vi "Initialiser caméra_CP.vi"(8 "entrée d'erreur (pas d'erreur)":errorcluster) -> (0 "sortie d'erreur":errorcluster, 2 "Camera":refnum<class "Camera.lvclass">, 3 "Buffer en sortie":refnum<class "Buffer.lvclass">, 4 "Devices":T1[](array[typedef]), 5 "Pixel Formats":string[](array[string]), 7 "Pixel Format":string)   [LabVIEW 2026]
uses:
  <vilib>/Serenial/G Industrial Camera/g_industrial_cam/Device Enumeration.ctl
  <vilib>/Serenial/G Industrial Camera/g_industrial_cam/Camera/Camera.lvclass
  <vilib>/Serenial/G Industrial Camera/g_industrial_cam/Buffer/Buffer.lvclass
  <vilib>/Serenial/G Industrial Camera/g_industrial_cam/Camera/Camera.lvclass/Camera.ctl
  <vilib>/Serenial/G Industrial Camera/g_industrial_cam/Buffer/Buffer.lvclass/Buffer.ctl
  <vilib>/Serenial/G Industrial Camera/g_industrial_cam/Camera/GetSetPixelFormat.vi
  <vilib>/Serenial/G Industrial Camera/g_industrial_cam/Camera/Check Not Disconnected.vi
  <vilib>/Utility/error.llb/Error Cluster From Error Code.vi
  <vilib>/Serenial/G Industrial Camera/g_industrial_cam/Camera/Destroy Stream Events.vi
  <vilib>/Serenial/G Industrial Camera/g_industrial_cam/g_industrial_cam.lvlib
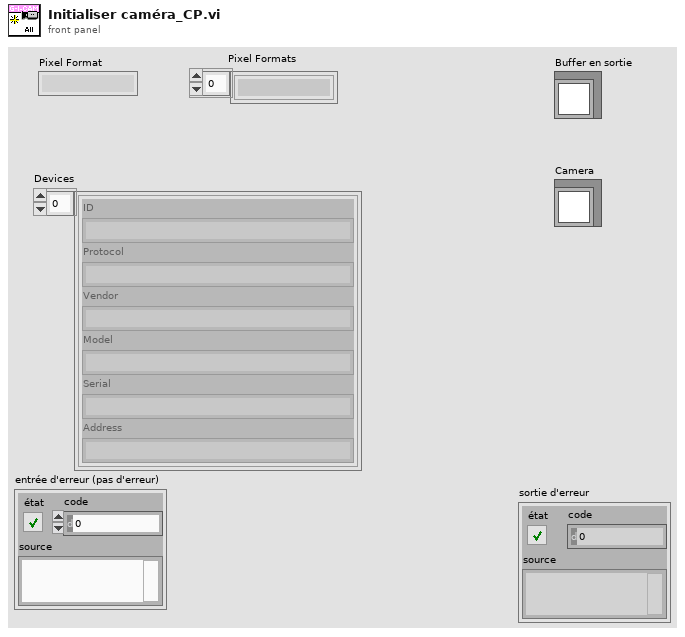
[diagram p1: front panel]
types:
  T1 = typedef "g_industrial_cam.lvlib/Device Enumeration.ctl" = cluster{"ID":string, "Protocol":string, "Vendor":string, "Model":string, "Serial":string, "Address":string}
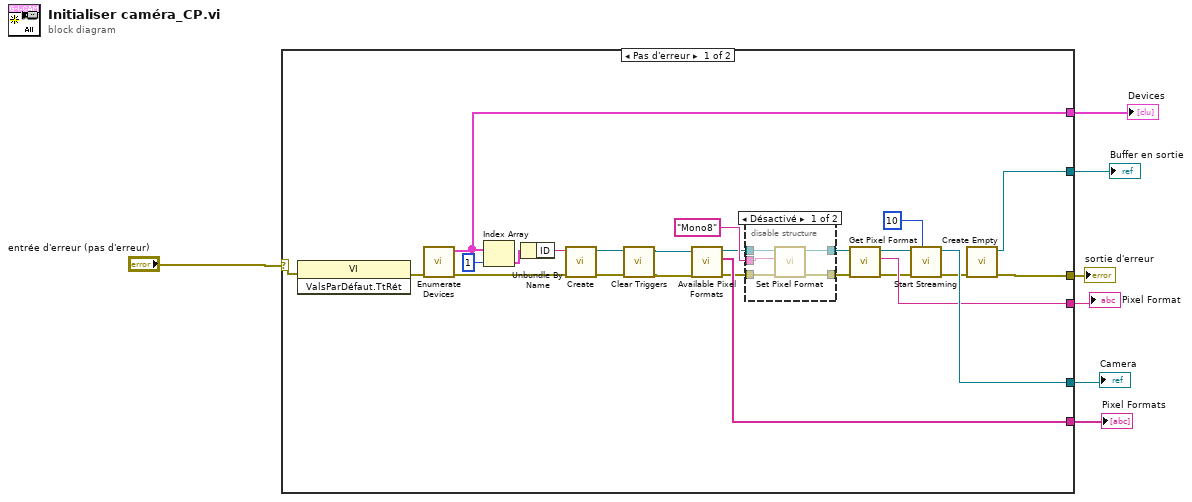
[diagram p0: block diagram]
diagram:
  n1 = case shown="Pas d'erreur" "entrée d'erreur (pas d'erreur)" {
    selector: "entrée d'erreur (pas d'erreur)" -> [w9 w40]
    tunnel: [w32 _] -> w7
    tunnel: [w28 _] -> w6
    tunnel: [w20 _] -> w5
    tunnel: [w18 _] -> w4
    tunnel: [w15 _] -> w3
    tunnel: [w14 w40] -> w2
    frame No Error {
      n2 = invoke class="VI" method="ValsParDéfaut.TtRét"(error in=w9) -> (error out=w25:errorcluster)  [unwired: 2 in, 2 out]
      n3 = call <vilib>:"Enumerate Devices.vi"("error in (no error)"=w25) -> ("error out"=w11:errorcluster, "Devices"=w32:T1[])  [unwired: 9 in]
      n4 = Index Array(array=w32, index=1 ("indice")) -> (element=w10:T1)
      n5 = Unbundle By Name(w10) -> ("ID"=w12:string)
      n6 = call <vilib>:"Create.vi"("error in (no error)"=w11, "Identifier (ID, IP etc)"=w12) -> ("error out"=w27:errorcluster, "Camera"=w26:refnum<class "Camera.lvclass">)  [unwired: 8 in]
      n7 = call <vilib>:"Clear Triggers.vi"("error in (no error)"=w27, "Camera in"=w26) -> ("error out"=w31:errorcluster, "Camera"=w30:refnum<class "Camera.lvclass">)  [unwired: 8 in]
      n8 = call <vilib>:"Available Pixel Formats.vi"("error in (no error)"=w31, "Camera in"=w30) -> ("error out"=w19:errorcluster, "Pixel Formats"=w20:string[], "Camera"=w22:refnum<class "Camera.lvclass">)  [unwired: 7 in]
      n9 = disable-structure shown="Désactivé" {
        disable-tunnel: w19 -> [w37 w38]
        disable-tunnel: [w36 w38] -> w21
        disable-tunnel: w22 -> [w35 w39]
        disable-tunnel: [w34 w39] -> w23
        disable-tunnel: "Mono8" ("Pixel Format") -> [w33 _]
        frame Disabled {
          n10 = call <vilib>:"Set Pixel Format.vi"("error in (no error)"=w37, "Pixel Format"=w33, "Camera in"=w35) -> ("error out"=w36:errorcluster, "Camera"=w34:refnum<class "Camera.lvclass">)  [unwired: 7 in]
        }
        frame Enabled {
        }
      }
      n11 = call <vilib>:"Get Pixel Format.vi"("error in (no error)"=w21, "Camera in"=w23) -> ("error out"=w16:errorcluster, "Pixel Format"=w18:string, "Camera"=w17:refnum<class "Camera.lvclass">)  [unwired: 7 in]
      n12 = call <vilib>:"Start Streaming.vi"("Additional Buffers (Default: 3)"=u16 10, "error in (no error)"=w16, "Camera in"=w17) -> ("error out"=w13:errorcluster, "Camera"=w28:refnum<class "Camera.lvclass">)  [unwired: 7 in]
      n13 = call <vilib>:"Create Empty.vi"("error in (no error)"=w13) -> ("error out"=w14:errorcluster, "Empty Buffer"=w15:refnum<class "Buffer.lvclass">)  [unwired: 9 in]
    }
    frame Error {
    }
  }
  "Devices" <- w7
  "Pixel Formats" <- w5
  "Camera" <- w6
  "Pixel Format" <- w4
  "Buffer en sortie" <- w3
  "sortie d'erreur" <- w2
